vi "VNA_Easy_Data2.vi"(1 "format (0 : log mag)":u16(ring) items=["log magnitude", "phase", "delay", "Smith chart", "polar", "linear magnitude", "standing wave ratio", "real", "imaginary"], 4 "CW freq (Hz)":dbl=1000.0 format="%.2e", 6 "sweep time (sec)":dbl=0.1 format="%.2f", 7 "sweep type (0 : linear)":u16(ring) items=["linear sweep", "logarithmic sweep", "frequency list", "CW time sweep", "power sweep"], 8 "error in (no error)":errorcluster, 9 "num points":u16(ring)=5 items=["3", "11", "21 ('20) / 26 ('53)", "51", "101", "201", "401", "801", "1601"], 10 "measurement (0 : S11)":u16(ring) items=["Ref1 : Forward S11 (A/R)", "Trans: Forward S21 (B/R)", "Trans: Reverse S12 (A/R)", "Ref1: Reverse S22 (B/R)", "Analog In, AUX input", "A/R", "B/R", "A/B", "A", "B", "R"], 11 "VISA Refnum in":refnum<visa-resource-name>) -> (0 "error out":errorcluster, 2 "Data":cluster{dbl[], sgl[]}, 3 "VISA Refnum out":refnum<visa-resource-name>)   [LabVIEW 2020]
uses:
  <instrlib>/Agilent 87XX Series/Agilent 87XX Series.lvlib
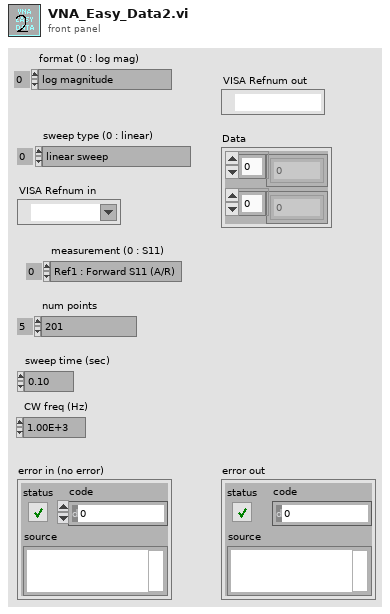
[diagram p1: front panel]
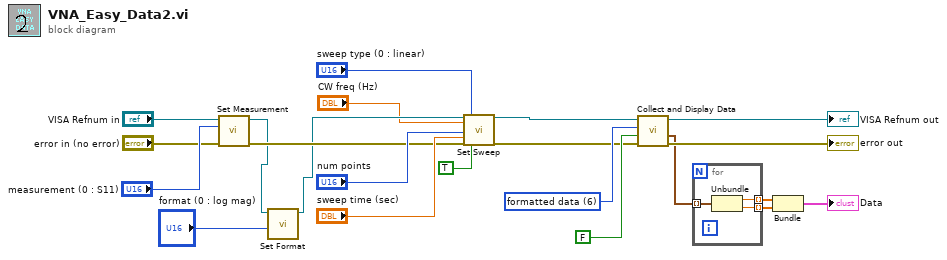
[diagram p0: block diagram]
diagram:
  w16 = u16 6 items=["raw data array 1", "raw data array 2", "raw data array 3", "raw data array 4", "error-corrected data", "error-corrected trace memory", "formatted data", "formatted memory", "formatted data / memory", "formatted data - memory"] ("data type (6 : formatted data)")
  n1 = call <instrlib>:"Set Measurement.vi"("error in (no error)"="error in (no error)", "measurement (0 : S11)"="measurement (0 : S11)", "VISA resource name"="VISA Refnum in") -> ("error out"=w5:errorcluster, "VISA resource name out"=w4:refnum<visa-resource-name>)  [unwired: 7 in]
  n2 = call <instrlib>:"Set Format.vi"("format (0 : log mag)"="format (0 : log mag)", "VISA resource name"=w4) -> ("VISA resource name out"=w3:refnum<visa-resource-name>)  [unwired: 8 in, 1 out]
  n3 = call <instrlib>:"Set Sweep.vi"("VISA resource name"=w3, "CW freq (Hz)"="CW freq (Hz)", "num points"="num points", "sweep time (sec)"="sweep time (sec)", "error in (no error)"=w5, "sweep type (0 : linear)"="sweep type (0 : linear)", "t: start/stop  f: center/span"=TRUE) -> ("VISA resource name out"=w8:refnum<visa-resource-name>, "error out"=w7:errorcluster)  [unwired: 11 in]
  n4 = call <instrlib>:"Collect and Display Data.vi"("error in (no error)"=w7, "save to file"=FALSE, "data type (6 : formatted data)"=w16, "VISA resource name"=w8) -> ("error out"=→"error out":errorcluster, "data values"=w13:cluster{"real / stim":dbl, "imag / resp":sgl}[], "VISA resource name out"=→"VISA Refnum out":refnum<visa-resource-name>)  [unwired: 4 in, 1 out]
  n5 = for {
    tunnel: w13 -> [w25] mode=indexing
    tunnel: [w24] -> w14 mode=indexing
    tunnel: [w23] -> w15 mode=indexing
    n6 = Unbundle(w25) -> ("real / stim"=w24:dbl, "imag / resp"=w23:sgl)
  }
  n7 = Bundle(w14, w15) -> (→"Data":cluster{dbl[], sgl[]})  [unwired: 1 in]
